vi "FGVScanWaveform.vi"(7 "Enum":T3, 8 "error in":errorcluster, 9 "scanWaveFormCtl In":T2={"slowWavePts"=1024, "fastWavePts"=1024, "slowWaveType"=enum."Triangle", "fastWaveType"=enum."Rounded", "slowRoundPts"=8, "fastRoundPts"=32, "singleDirectionScan"=TRUE}) -> (0 "error out":errorcluster, 1 "scanWaveFormCtl Out":T2={"slowWavePts"=1024, "fastWavePts"=1024, "slowWaveType"=enum."Triangle", "fastWaveType"=enum."Rounded", "slowRoundPts"=8, "fastRoundPts"=32, "singleDirectionScan"=TRUE})   [LabVIEW 2016]
uses:
  controls/Enum.ctl
  controls/ScanWaveform.ctl
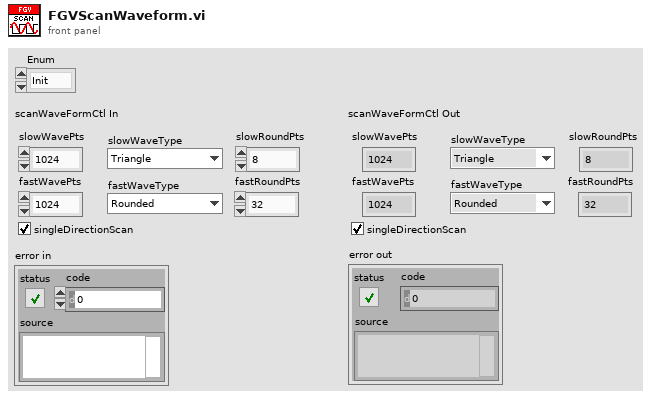
[diagram p1: front panel]
types:
  T1 = typedef "ScanWaveform.ctl" = enum16{"Sine", "Triangle", "Rounded"}
  T2 = cluster{"slowWavePts":u16, "fastWavePts":u16, "slowWaveType":T1, "fastWaveType":T1, "slowRoundPts":u16, "fastRoundPts":u16, "singleDirectionScan":bool}
  T3 = typedef "Enum.ctl" = enum16{"Init", "Read", "Write"}
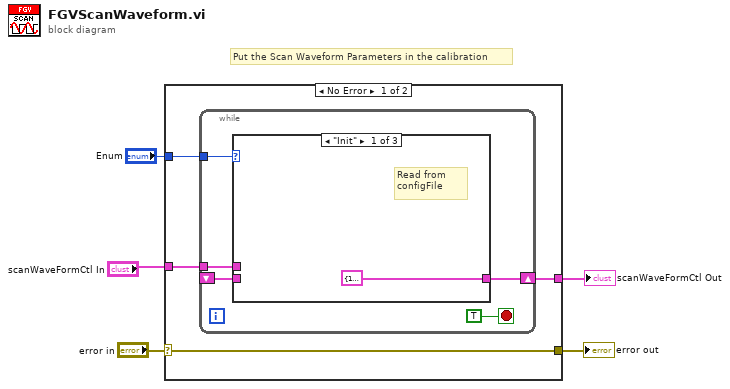
[diagram p0: block diagram]
diagram:
  # "Put the Scan Waveform Parameters in the calibration"
  n1 = case shown="No Error" "error in" {
    selector: "error in" -> [w8 w19]
    tunnel: "Enum" -> [w9 _]
    tunnel: [w8 w19] -> w4
    tunnel: "scanWaveFormCtl In" -> [w7 w18]
    tunnel: [w6 w18] -> w1
    frame No Error {
      n2 = while {
        tunnel: w9 -> [w13]
        tunnel: w7 -> [w12]
        shift-right: [w11] -> w6
        shift-left: _ -> [w10]
        stop <- TRUE stop-if-true
        n3 = case shown="\"Init\"" w13 {
          tunnel: w12 -> [_ _ w17]
          tunnel: [T2 {"slowWavePts"=1024, "fastWavePts"=1024, "slowWaveType"=enum."Triangle", "fastWaveType"=enum."Rounded", "slowRoundPts"=8, "fastRoundPts"=32, "singleDirectionScan"=TRUE} ("scanWaveFormCtl In") w16 w17] -> w11
          tunnel: w10 -> [_ w16 _]
          frame "Init" {
            # "Read from configFile"
          }
          frame "Read", Default {
          }
          frame "Write" {
          }
        }
      }
    }
    frame Error {
    }
  }
  "error out" <- w4
  "scanWaveFormCtl Out" <- w1
